vi "Results FGV.vi"(6 "Method":T1, 8 "error in":errorcluster, 11 "Water Tunnel Results in":refnum<class "Water Tunnel Results.lvclass">) -> (0 "error out":errorcluster, 3 "Water Tunnel  Results out":refnum<class "Water Tunnel Results.lvclass">)   [LabVIEW 2019, in "Results.lvlib" / "Water Tunnel Results.lvclass"]
uses:
  Water Tunnel Results.lvclass
  Results Method.ctl
  Results.lvlib
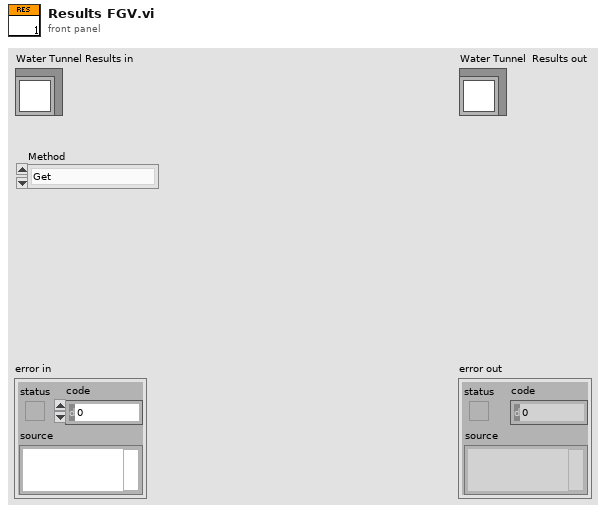
[diagram p1: front panel]
types:
  T1 = typedef "Results.lvlib/Results Method.ctl" = enum16{"Get", "Set"}
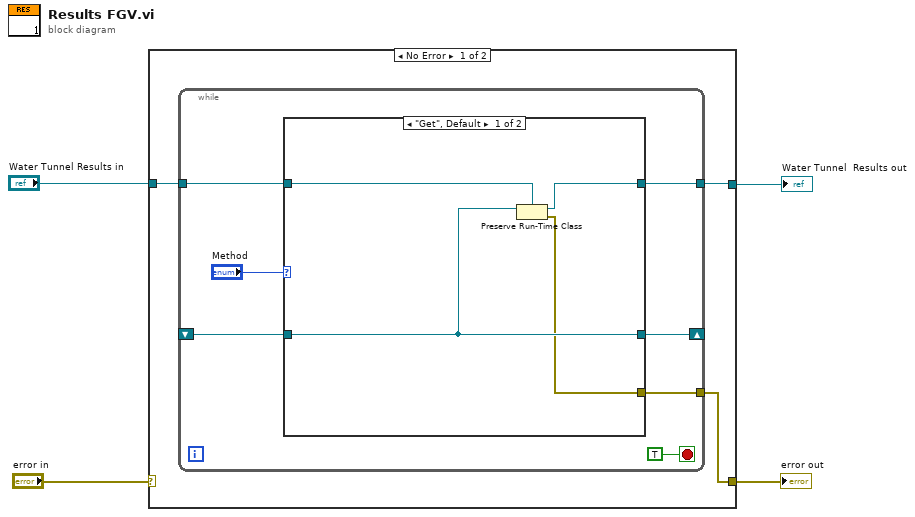
[diagram p0: block diagram]
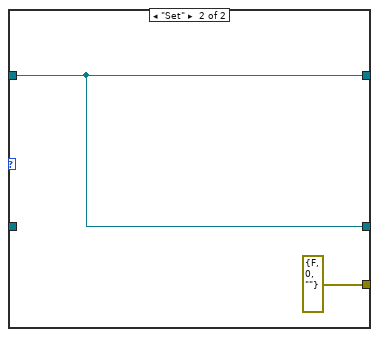
[diagram p2: hidden frame]
diagram:
  n1 = case shown="No Error" "error in" {
    selector: "error in" -> [_ w22]
    tunnel: [w5 w22] -> w3
    tunnel: "Water Tunnel Results in" -> [w7 w21]
    tunnel: [w6 w21] -> w2
    frame No Error {
      n2 = while {
        tunnel: w7 -> [w14]
        tunnel: [w13] -> w6
        shift-right: [w11] -> _
        shift-left: _ -> [w10]
        tunnel: [w8] -> w5
        stop <- TRUE stop-if-true
        n3 = case shown="\"Get\", Default" "Method" {
          tunnel: w14 -> [w17 w20]
          tunnel: [w18 w20] -> w11
          tunnel: [w16 w20] -> w13
          tunnel: w10 -> [w18 _]
          tunnel: [w15 errorcluster {"status"=FALSE, "code"=0, "source"=""} ("error out")] -> w8
          frame "Get", Default {
            n4 = Preserve Run-Time Class(object in=w18, 2:w17) -> (object out=w16:refnum<class "Water Tunnel Results.lvclass">, error out=w15:errorcluster)  [unwired: 1 in]
          }
          frame "Set" {
          }
        }
      }
    }
    frame Error {
    }
  }
  "error out" <- w3
  "Water Tunnel  Results out" <- w2
